vi "Event Login.vi"(8 "error in (no error)":errorcluster, 11 "[V] Login in":refnum<class "[V] Login.lvclass">) -> (0 "error out":errorcluster, 3 "[V] Login out":refnum<class "[V] Login.lvclass">)   [LabVIEW 2020, in "[V] Login.lvlib" / "[V] Login.lvclass"]
uses:
  [V] Login.lvclass
  [V] Login.lvclass/[V] Login.ctl
  INF of [V] Login Messages/Login Request Msg/Login Request Msg.lvclass/Login Request Msg.ctl
  <vilib>/ActorFramework/Message Enqueuer/Message Enqueuer.lvclass/Message Enqueuer.ctl
  <vilib>/ActorFramework/Message Enqueuer/Enqueue.vi
  INF of [V] Login Messages/Login Request Msg/Login Request Msg.lvclass
  C:/Program Files/National Instruments/LabVIEW 2020/vi.lib/ActorFramework/Message/Message.lvclass
  <vilib>/ActorFramework/Message Priority Queue/Priority Enqueue.vi
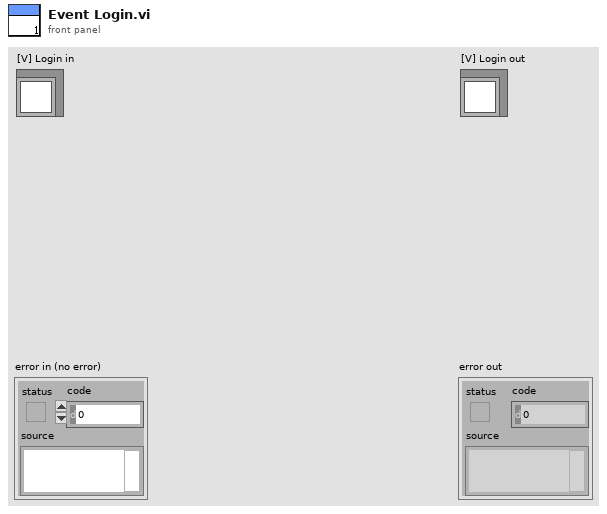
[diagram p1: front panel]
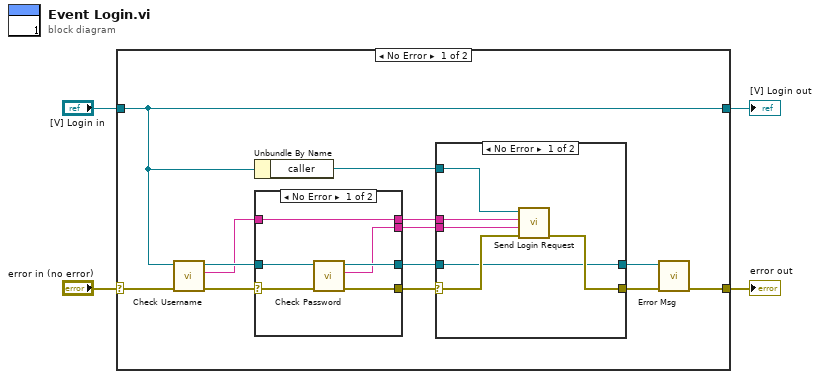
[diagram p0: block diagram]
diagram:
  n1 = case shown="No Error" "error in (no error)" {
    selector: "error in (no error)" -> [w17 w36]
    tunnel: [w7 w36] -> w3
    tunnel: [w6 w35] -> w1
    tunnel: "[V] Login in" -> [w6 w35]
    frame No Error {
      n2 = call "Check Username.vi"("error in (no error)"=w17, "[V] Login in"=w6) -> ("error out"=w16:errorcluster, "username"=w14:string, "[V] Login out"=w15:refnum<class "[V] Login.lvclass">)  [unwired: 7 in]
      n3 = Unbundle By Name(w6) -> ("caller"=w5:refnum<class "Message Enqueuer.lvclass">)
      n4 = case shown="No Error" w16 {
        selector: w16 -> [w31 w34]
        tunnel: [w29 w34] -> w10
        tunnel: w15 -> [w30 w33]
        tunnel: [w28 w33] -> w11
        tunnel: w14 -> [w27 w32]
        tunnel: [w27 w32] -> w13
        tunnel: [w26 _] -> w12
        frame No Error {
          n5 = call "Check Password.vi"("error in (no error)"=w31, "[V] Login in"=w30) -> ("error out"=w29:errorcluster, "password"=w26:string, "[V] Login out"=w28:refnum<class "[V] Login.lvclass">)  [unwired: 7 in]
        }
        frame Error {
        }
      }
      n6 = case shown="No Error" w10 {
        selector: w10 -> [w23 w25]
        tunnel: w13 -> [w20 _]
        tunnel: w12 -> [w21 _]
        tunnel: w11 -> [w19 w24]
        tunnel: [w22 w25] -> w8
        tunnel: [w19 w24] -> w9
        tunnel: w5 -> [w18 _]
        frame No Error {
          n7 = call "Send Login Request.vi"("error in (no error)"=w23, "password"=w21, "username"=w20, "Message Enqueuer"=w18) -> ("error out"=w22:errorcluster)  [unwired: 6 in, 1 out]
        }
        frame Error {
        }
      }
      n8 = call "Error Msg.vi"("error in (no error)"=w8, "[V] Login in"=w9) -> ("error out"=w7:errorcluster)  [unwired: 8 in, 1 out]
    }
    frame Error {
    }
  }
  "error out" <- w3
  "[V] Login out" <- w1
